vi "RT Encode.vi"(7 "Reset":bool, 10 "B":bool, 11 "A":bool) -> (3 "Encode":dbl)   [LabVIEW 2017]
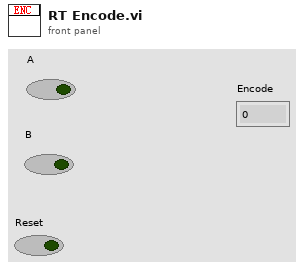
[diagram p1: front panel]
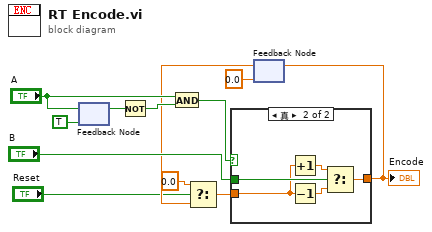
[diagram p0: block diagram]
diagram:
  n1 = feedback #1(TRUE ("布尔")) -> (w11:bool)
  n2 = feedback-in #1("A") -> ()
  n3 = Not(x=w11) -> (.not. x?=w10:bool)
  n4 = And(x="A", y=w10) -> (x .and. y?=w7:bool)
  n5 = feedback #2(0.0) -> (w5:dbl)
  n6 = Select(t=0.0, s="Reset", f=w5) -> (s? t:f=w3:dbl)
  n7 = case shown="真" w7 {
    tunnel: "B" -> [_ w18]
    tunnel: w3 -> [w13 w14]
    tunnel: [w13 w15] -> w6
    frame False {
    }
    frame True {
      n8 = Increment(x=w14) -> (x+1=w17:dbl)
      n9 = Decrement(x=w14) -> (x-1=w16:dbl)
      n10 = Select(t=w17, s=w18, f=w16) -> (s? t:f=w15:dbl)
    }
  }
  "Encode" <- w6
  n11 = feedback-in #2(w6) -> ()
